vi "MAIN.vi"() -> ()   [LabVIEW 2017]
uses:
  Main Control Functions.ctl
  TableType.ctl
  <vilib>/Utility/file.llb/Write Delimited Spreadsheet (DBL).vi
  <vilib>/Utility/file.llb/Read Delimited Spreadsheet (DBL).vi
panel:
  in  "Start":bool
  in  "Listbox":i32(listbox)
  in  "Stop":bool
  out "Time":string caption="String"
  in  "String":string
  in  "Tab Control":enum32{"Page 1", "Page 2"}(tab)
  in  "Voltage":dbl caption="Numeric"
  in  "Day Code":string caption="String"
  in  "Unit ID":i32 caption="Numeric"
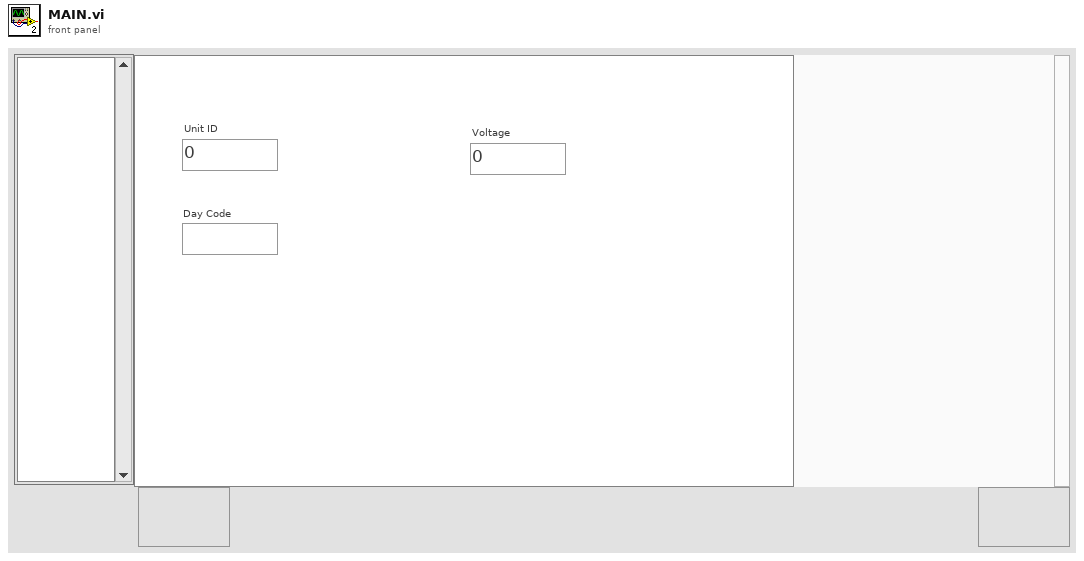
[diagram p1: front panel]
types:
  T1 = typedef "Main Control Functions.ctl" = enum16{"Initialize", "Wait", "Read PN Wfm", "Read SP Wfm", "Read FrHz Wfm", "Read FrHzV Wfm", "Read Power Wfm", "Read Curr Wfm", "Check Q", "Exit"}
  T2 = typedef "TableType.ctl" = enum16{"PhaseNoise", "Spectrum", "FreqHz", "FreqHzV", "Power", "Current"}
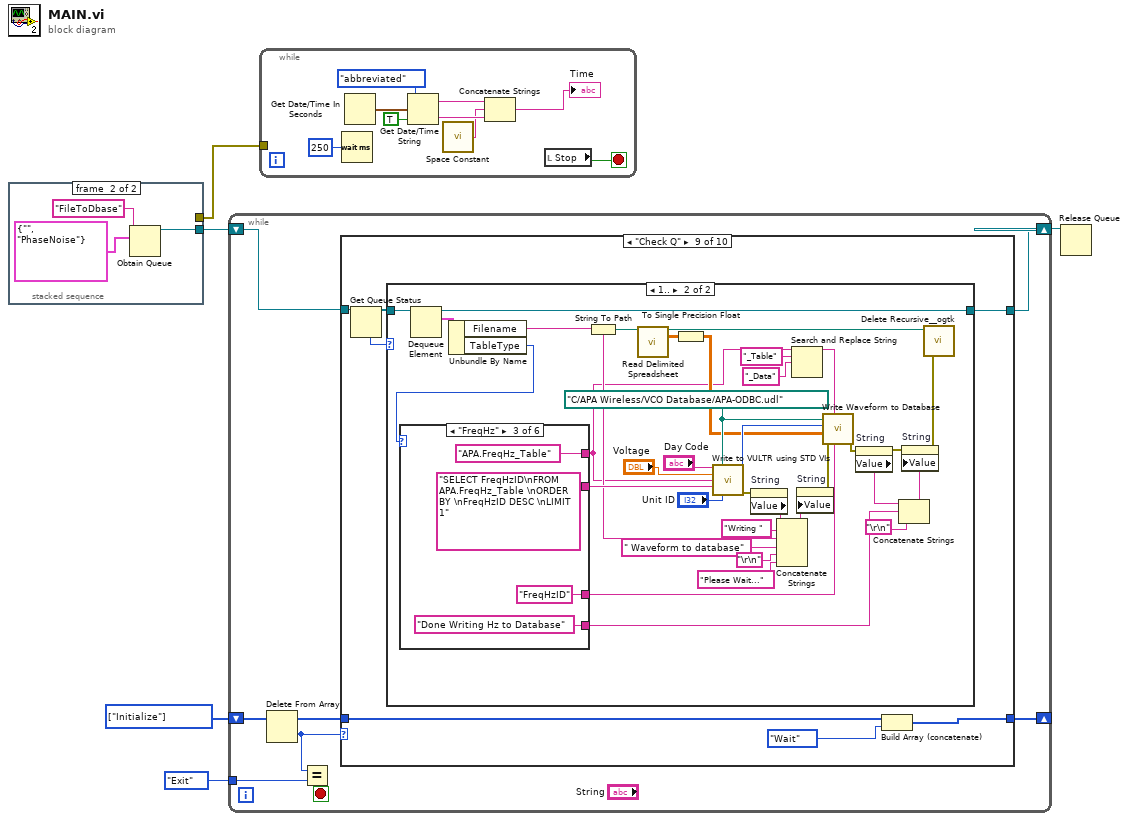
[diagram p0: block diagram]
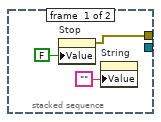
[diagram p2: hidden frame]
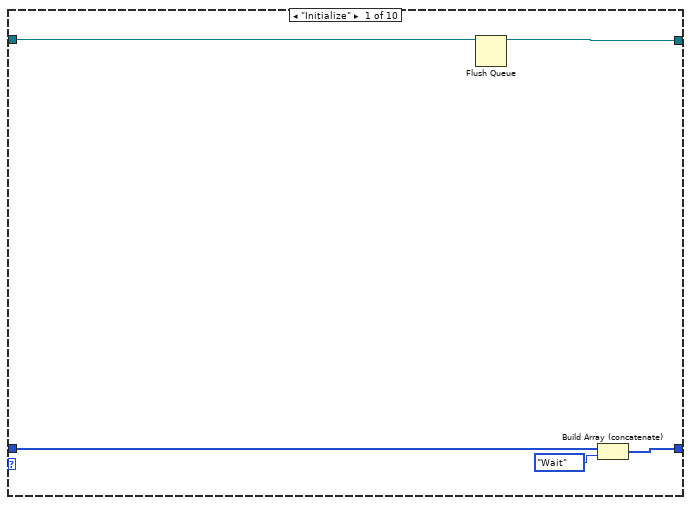
[diagram p3: hidden frame]
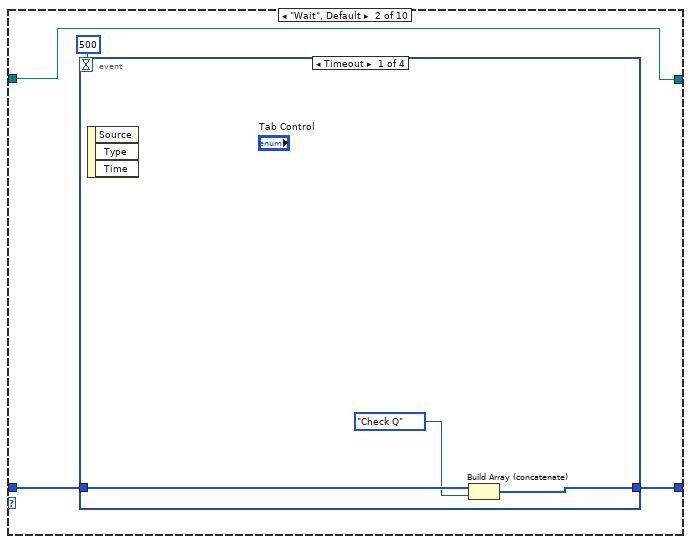
[diagram p4: hidden frame]
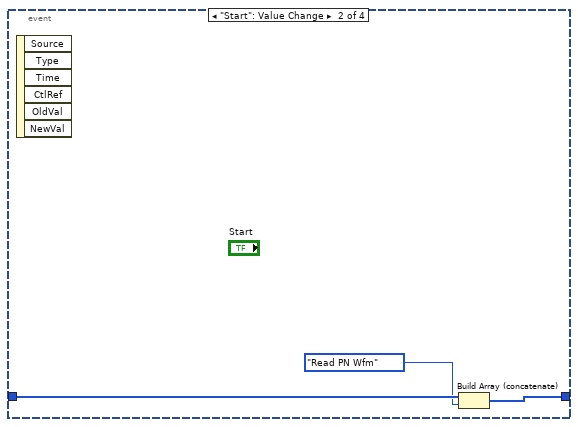
[diagram p5: hidden frame]
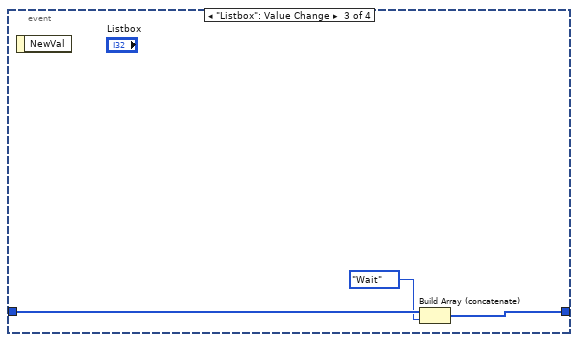
[diagram p6: hidden frame]
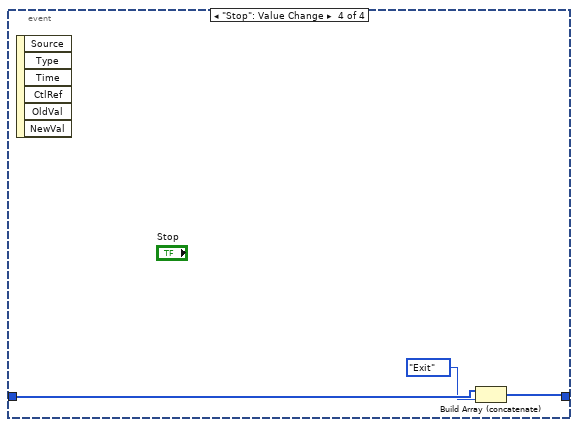
[diagram p7: hidden frame]
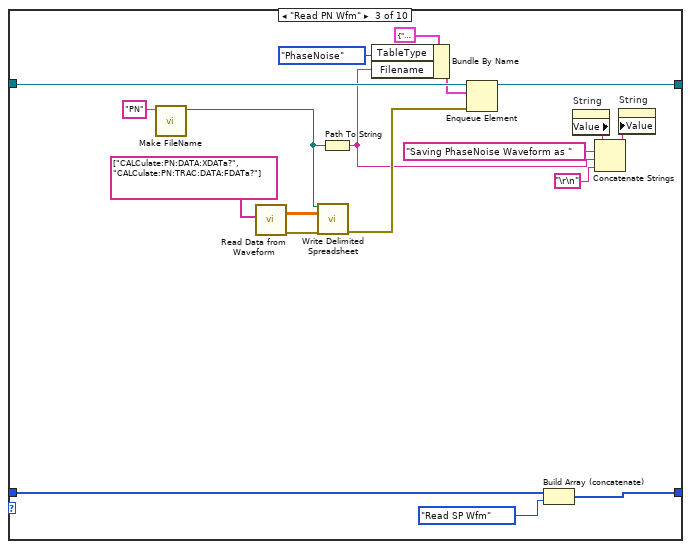
[diagram p8: hidden frame]
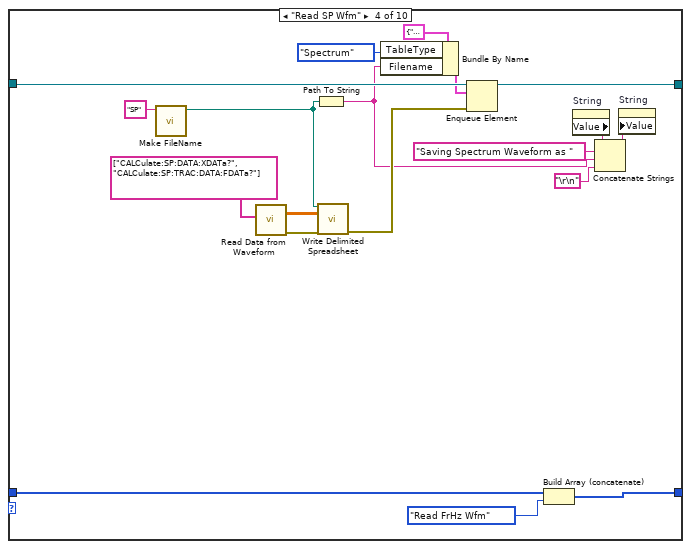
[diagram p9: hidden frame]
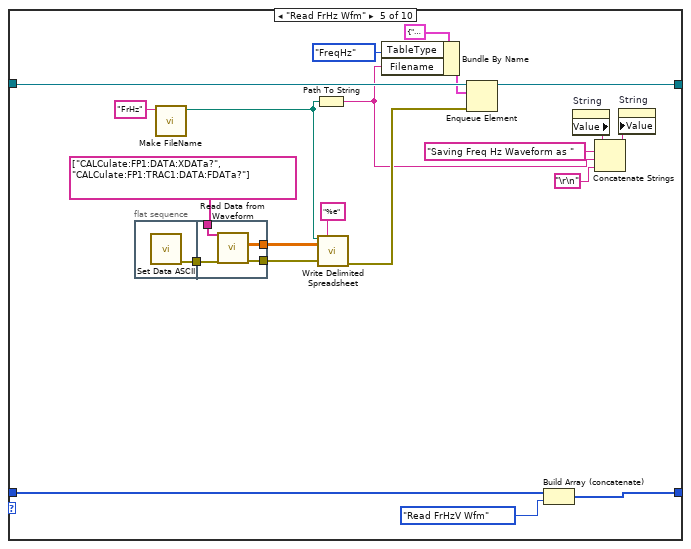
[diagram p10: hidden frame]
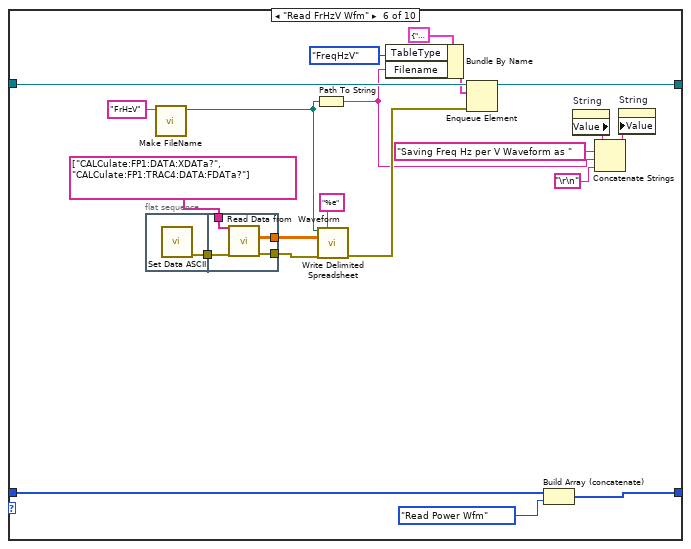
[diagram p11: hidden frame]
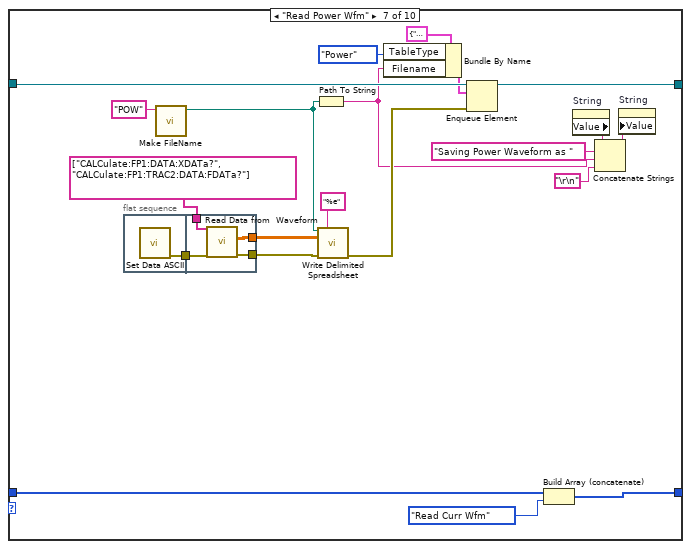
[diagram p12: hidden frame]
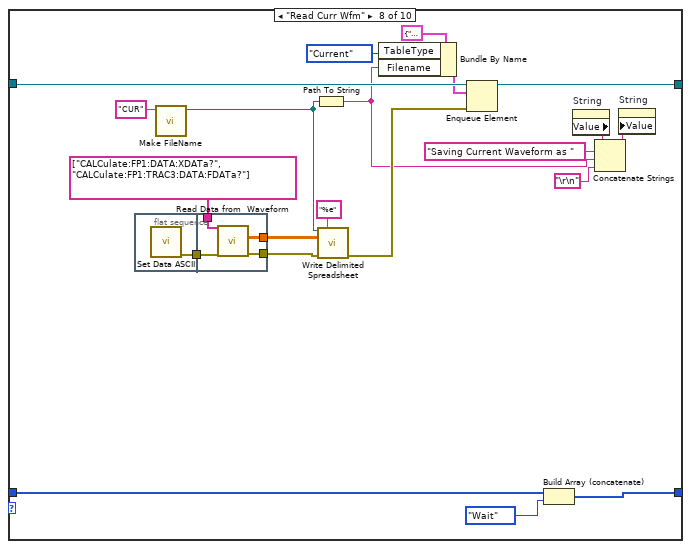
[diagram p13: hidden frame]
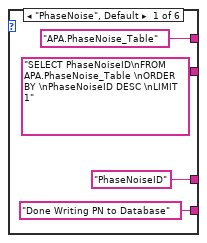
[diagram p15: hidden frame]
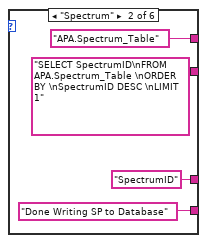
[diagram p16: hidden frame]
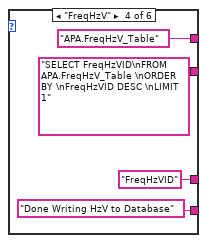
[diagram p17: hidden frame]
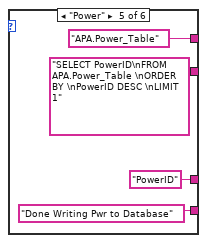
[diagram p18: hidden frame]
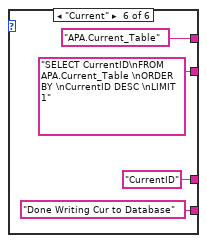
[diagram p19: hidden frame]
diagram:
  w1 = T1[] [enum."Initialize"] items=["Initialize", "Wait", "Read PN Wfm", "Read SP Wfm", "Read FrHz Wfm", "Read FrHzV Wfm", "Read Power Wfm", "Read Curr Wfm", "Check Q", "Exit"]
  n1 = stacked-sequence {
    tunnel: [_ w10] -> w3
    tunnel: [w8 _] -> w2
    frame #0 {
      n2 = property on="Stop" class="Bool (strict)"("Value"=FALSE ("Stop")) -> (error out=w8:errorcluster)  [unwired: 2 in, 1 out]
      n3 = property on="String" class="Str"("Value"="") -> ()  [unwired: 2 in, 2 out]
    }
    frame #1 {
      n4 = Obtain Queue(name (unnamed)="FileToDbase", element data type=cluster{"Filename":string, "TableType":T2} {"Filename"="", "TableType"=enum."PhaseNoise"}) -> (queue out=w10:refnum<queue>)  [unwired: 3 in, 2 out]
    }
  }
  n5 = while {
    shift-right: [w14] -> _
    shift-left: w1 -> [w17]
    tunnel: Main_Control_Functions."Exit" ("Enum") -> [w19]
    shift-right: [w12] -> w4
    shift-left: w3 -> [w13]
    stop <- w18 stop-if-true
    n6 = Delete From Array(array=w17) -> (deleted portion=w16:T1, array with subset deleted=w15:T1[])  [unwired: 2 in]
    n7 = Equal?(x=w16, y=w19) -> (x = y?=w18:bool)
    n8 = case shown="\"Check Q\"" w16 {
      tunnel: w15 -> [w24 w28 w52 w71 w95 w121 w147 w173 w189 w251]
      tunnel: [w22 w27 w47 w66 w90 w116 w142 w168 w185 w251] -> w14
      tunnel: w13 -> [w21 w26 w55 w74 w98 w124 w150 w176 w188 w250]
      tunnel: [w20 w26 w54 w73 w97 w123 w149 w175 w186 w250] -> w12
      frame "Initialize" {
        n9 = Flush Queue(queue=w21) -> (queue out=w20:refnum<queue>)  [unwired: 1 in, 2 out]
        n10 = Build Array (concatenate)(w24, Main_Control_Functions."Wait" ("Enum")) -> (w22:T1[])
      }
      frame "Wait", Default {
        n11 = event shown="[0] Timeout" {
          selector: _ -> [_ _ _ _]
          dyn-events: _ -> [_ _ _ _]
          timeout: 500 -> [_ _ _ _]
          tunnel: [w30 w33 w36 w39] -> w27
          tunnel: w28 -> [w31 w34 w37 w40]
          event Timeout {
            n12 = event-data() -> ()  [unwired: 1 in, 3 out]
            n13 = Build Array (concatenate)(w31, Main_Control_Functions."Check Q" ("Enum")) -> (w30:T1[])
          }
          event "Start": Value Change {
            n14 = event-data() -> ()  [unwired: 1 in, 6 out]
            n15 = Build Array (concatenate)(w34, Main_Control_Functions."Read PN Wfm" ("Enum")) -> (w33:T1[])
          }
          event "Listbox": Value Change {
            n16 = event-data() -> ()  [unwired: 1 in, 1 out]
            n17 = Build Array (concatenate)(w37, Main_Control_Functions."Wait" ("Enum")) -> (w36:T1[])
          }
          event "Stop": Value Change {
            n18 = event-data() -> ()  [unwired: 1 in, 6 out]
            n19 = Build Array (concatenate)(w40, Main_Control_Functions."Exit" ("Enum")) -> (w39:T1[])
          }
        }
      }
      frame "Read PN Wfm" {
        n20 = call "Make FileName.vi"("Meas Name"="PN") -> ("Path"=w56:path)  [unwired: 10 in]
        n21 = call "Read Data from  Waveform.vi"("Commands"=string[] ["CALCulate:PN:DATA:XDATa?", "CALCulate:PN:TRAC:DATA:FDATa?"]) -> ("error out"=w58:errorcluster, "Results"=w57:sgl[][])  [unwired: 9 in]
        n22 = call-poly <vilib>:"Write Delimited Spreadsheet.vi"("file path (dialog if empty)"=w56, "2D data"=w57, "error in (no error)"=w58) -> ("error out"=w53:errorcluster)  [unwired: 11 in, 1 out]
        n23 = Path To String(path=w56) -> (string=w43:string)
        n24 = Bundle By Name(cluster=cluster{"Filename":string, "TableType":T2} {"Filename"="", "TableType"=enum."PhaseNoise"} ("element"), "TableType"=TableType."PhaseNoise", "Filename"=w43) -> (w41:cluster{"Filename":string, "TableType":T2})
        n25 = Enqueue Element(queue=w55, element=w41, error in (no error)=w53) -> (queue out=w54:refnum<queue>)  [unwired: 1 in, 2 out]
        n26 = Build Array (concatenate)(w52, Main_Control_Functions."Read SP Wfm" ("Enum")) -> (w47:T1[])
        n27 = property on="String" class="Str"() -> ("Value"=w50:string)  [unwired: 2 in, 2 out]
        n28 = Concatenate Strings(w50, "Saving PhaseNoise Waveform as " ("string"), w43, "\r\n") -> (w51:string)
        n29 = property on="String" class="Str"("Value"=w51) -> ()  [unwired: 2 in, 2 out]
      }
      frame "Read SP Wfm" {
        n30 = call "Make FileName.vi"("Meas Name"="SP") -> ("Path"=w75:path)  [unwired: 10 in]
        n31 = call "Read Data from  Waveform.vi"("Commands"=string[] ["CALCulate:SP:DATA:XDATa?", "CALCulate:SP:TRAC:DATA:FDATa?"]) -> ("error out"=w77:errorcluster, "Results"=w76:sgl[][])  [unwired: 9 in]
        n32 = Path To String(path=w75) -> (string=w61:string)
        n33 = call-poly <vilib>:"Write Delimited Spreadsheet.vi"("file path (dialog if empty)"=w75, "2D data"=w76, "error in (no error)"=w77) -> ("error out"=w72:errorcluster)  [unwired: 11 in, 1 out]
        n34 = Bundle By Name(cluster=cluster{"Filename":string, "TableType":T2} {"Filename"="", "TableType"=enum."PhaseNoise"} ("element"), "TableType"=TableType."Spectrum", "Filename"=w61) -> (w60:cluster{"Filename":string, "TableType":T2})
        n35 = Enqueue Element(queue=w74, element=w60, error in (no error)=w72) -> (queue out=w73:refnum<queue>)  [unwired: 1 in, 2 out]
        n36 = Build Array (concatenate)(w71, Main_Control_Functions."Read FrHz Wfm" ("Enum")) -> (w66:T1[])
        n37 = property on="String" class="Str"() -> ("Value"=w69:string)  [unwired: 2 in, 2 out]
        n38 = Concatenate Strings(w69, "Saving Spectrum Waveform as " ("string"), w61, "\r\n") -> (w70:string)
        n39 = property on="String" class="Str"("Value"=w70) -> ()  [unwired: 2 in, 2 out]
      }
      frame "Read FrHz Wfm" {
        n40 = flat-sequence {
          tunnel: [w100] -> w87
          tunnel: w87 -> [w104]
          tunnel: string[] ["CALCulate:FP1:DATA:XDATa?", "CALCulate:FP1:TRAC1:DATA:FDATa?"] ("Commands") -> [w103]
          tunnel: [w102] -> w85
          tunnel: [w101] -> w84
          frame #0 {
            n41 = call "Set Data ASCII.vi"() -> ("error out"=w100:errorcluster)  [unwired: 11 in]
          }
          frame #1 {
            n42 = call "Read Data from  Waveform.vi"("error in (no error)"=w104, "Commands"=w103) -> ("error out"=w102:errorcluster, "Results"=w101:sgl[][])  [unwired: 8 in]
          }
        }
        n43 = call "Make FileName.vi"("Meas Name"="FrHz") -> ("Path"=w99:path)  [unwired: 10 in]
        n44 = Path To String(path=w99) -> (string=w79:string)
        n45 = call-poly <vilib>:"Write Delimited Spreadsheet.vi"("file path (dialog if empty)"=w99, "format (%.3f)"="%e", "2D data"=w84, "error in (no error)"=w85) -> ("error out"=w96:errorcluster)  [unwired: 10 in, 1 out]
        n46 = Bundle By Name(cluster=cluster{"Filename":string, "TableType":T2} {"Filename"="", "TableType"=enum."PhaseNoise"} ("element"), "TableType"=TableType."FreqHz", "Filename"=w79) -> (w80:cluster{"Filename":string, "TableType":T2})
        n47 = Enqueue Element(queue=w98, element=w80, error in (no error)=w96) -> (queue out=w97:refnum<queue>)  [unwired: 1 in, 2 out]
        n48 = Build Array (concatenate)(w95, Main_Control_Functions."Read FrHzV Wfm" ("Enum")) -> (w90:T1[])
        n49 = property on="String" class="Str"() -> ("Value"=w93:string)  [unwired: 2 in, 2 out]
        n50 = Concatenate Strings(w93, "Saving Freq Hz Waveform as " ("string"), w79, "\r\n") -> (w94:string)
        n51 = property on="String" class="Str"("Value"=w94) -> ()  [unwired: 2 in, 2 out]
      }
      frame "Read FrHzV Wfm" {
        n52 = flat-sequence {
          tunnel: [w126] -> w113
          tunnel: w113 -> [w130]
          tunnel: string[] ["CALCulate:FP1:DATA:XDATa?", "CALCulate:FP1:TRAC4:DATA:FDATa?"] ("Commands") -> [w129]
          tunnel: [w128] -> w110
          tunnel: [w127] -> w111
          frame #0 {
            n53 = call "Set Data ASCII.vi"() -> ("error out"=w126:errorcluster)  [unwired: 11 in]
          }
          frame #1 {
            n54 = call "Read Data from  Waveform.vi"("error in (no error)"=w130, "Commands"=w129) -> ("error out"=w128:errorcluster, "Results"=w127:sgl[][])  [unwired: 8 in]
          }
        }
        n55 = call "Make FileName.vi"("Meas Name"="FrHzV") -> ("Path"=w125:path)  [unwired: 10 in]
        n56 = Path To String(path=w125) -> (string=w105:string)
        n57 = call-poly <vilib>:"Write Delimited Spreadsheet.vi"("file path (dialog if empty)"=w125, "format (%.3f)"="%e", "2D data"=w111, "error in (no error)"=w110) -> ("error out"=w122:errorcluster)  [unwired: 10 in, 1 out]
        n58 = Bundle By Name(cluster=cluster{"Filename":string, "TableType":T2} {"Filename"="", "TableType"=enum."PhaseNoise"} ("element"), "TableType"=TableType."FreqHzV", "Filename"=w105) -> (w106:cluster{"Filename":string, "TableType":T2})
        n59 = Enqueue Element(queue=w124, element=w106, error in (no error)=w122) -> (queue out=w123:refnum<queue>)  [unwired: 1 in, 2 out]
        n60 = Build Array (concatenate)(w121, Main_Control_Functions."Read Power Wfm" ("Enum")) -> (w116:T1[])
        n61 = property on="String" class="Str"() -> ("Value"=w119:string)  [unwired: 2 in, 2 out]
        n62 = Concatenate Strings(w119, "Saving Freq Hz per V Waveform as " ("string"), w105, "\r\n") -> (w120:string)
        n63 = property on="String" class="Str"("Value"=w120) -> ()  [unwired: 2 in, 2 out]
      }
      frame "Read Power Wfm" {
        n64 = flat-sequence {
          tunnel: [w152] -> w139
          tunnel: w139 -> [w156]
          tunnel: string[] ["CALCulate:FP1:DATA:XDATa?", "CALCulate:FP1:TRAC2:DATA:FDATa?"] ("Commands") -> [w155]
          tunnel: [w154] -> w137
          tunnel: [w153] -> w138
          frame #0 {
            n65 = call "Set Data ASCII.vi"() -> ("error out"=w152:errorcluster)  [unwired: 11 in]
          }
          frame #1 {
            n66 = call "Read Data from  Waveform.vi"("error in (no error)"=w156, "Commands"=w155) -> ("error out"=w154:errorcluster, "Results"=w153:sgl[][])  [unwired: 8 in]
          }
        }
        n67 = call "Make FileName.vi"("Meas Name"="POW") -> ("Path"=w151:path)  [unwired: 10 in]
        n68 = Path To String(path=w151) -> (string=w131:string)
        n69 = call-poly <vilib>:"Write Delimited Spreadsheet.vi"("file path (dialog if empty)"=w151, "format (%.3f)"="%e", "2D data"=w138, "error in (no error)"=w137) -> ("error out"=w148:errorcluster)  [unwired: 10 in, 1 out]
        n70 = Bundle By Name(cluster=cluster{"Filename":string, "TableType":T2} {"Filename"="", "TableType"=enum."PhaseNoise"} ("element"), "TableType"=TableType."Power", "Filename"=w131) -> (w132:cluster{"Filename":string, "TableType":T2})
        n71 = Enqueue Element(queue=w150, element=w132, error in (no error)=w148) -> (queue out=w149:refnum<queue>)  [unwired: 1 in, 2 out]
        n72 = Build Array (concatenate)(w147, Main_Control_Functions."Read Curr Wfm" ("Enum")) -> (w142:T1[])
        n73 = property on="String" class="Str"() -> ("Value"=w145:string)  [unwired: 2 in, 2 out]
        n74 = Concatenate Strings(w145, "Saving Power Waveform as " ("string"), w131, "\r\n") -> (w146:string)
        n75 = property on="String" class="Str"("Value"=w146) -> ()  [unwired: 2 in, 2 out]
      }
      frame "Read Curr Wfm" {
        n76 = flat-sequence {
          tunnel: [w178] -> w165
          tunnel: w165 -> [w182]
          tunnel: string[] ["CALCulate:FP1:DATA:XDATa?", "CALCulate:FP1:TRAC3:DATA:FDATa?"] ("Commands") -> [w181]
          tunnel: [w180] -> w163
          tunnel: [w179] -> w164
          frame #0 {
            n77 = call "Set Data ASCII.vi"() -> ("error out"=w178:errorcluster)  [unwired: 11 in]
          }
          frame #1 {
            n78 = call "Read Data from  Waveform.vi"("error in (no error)"=w182, "Commands"=w181) -> ("error out"=w180:errorcluster, "Results"=w179:sgl[][])  [unwired: 8 in]
          }
        }
        n79 = call "Make FileName.vi"("Meas Name"="CUR") -> ("Path"=w177:path)  [unwired: 10 in]
        n80 = Path To String(path=w177) -> (string=w157:string)
        n81 = call-poly <vilib>:"Write Delimited Spreadsheet.vi"("file path (dialog if empty)"=w177, "format (%.3f)"="%e", "2D data"=w164, "error in (no error)"=w163) -> ("error out"=w174:errorcluster)  [unwired: 10 in, 1 out]
        n82 = Bundle By Name(cluster=cluster{"Filename":string, "TableType":T2} {"Filename"="", "TableType"=enum."PhaseNoise"} ("element"), "TableType"=TableType."Current", "Filename"=w157) -> (w158:cluster{"Filename":string, "TableType":T2})
        n83 = Enqueue Element(queue=w176, element=w158, error in (no error)=w174) -> (queue out=w175:refnum<queue>)  [unwired: 1 in, 2 out]
        n84 = Build Array (concatenate)(w173, Main_Control_Functions."Wait" ("Enum")) -> (w168:T1[])
        n85 = property on="String" class="Str"() -> ("Value"=w171:string)  [unwired: 2 in, 2 out]
        n86 = Concatenate Strings(w171, "Saving Current Waveform as " ("string"), w157, "\r\n") -> (w172:string)
        n87 = property on="String" class="Str"("Value"=w172) -> ()  [unwired: 2 in, 2 out]
      }
      frame "Check Q" {
        n88 = Get Queue Status(queue=w188) -> (queue out=w187:refnum<queue>, # elements in queue=w183:i32)  [unwired: 2 in, 6 out]
        n89 = case shown="1.." w183 {
          tunnel: w187 -> [w190 w225]
          tunnel: [w190 w220] -> w186
          frame ..0 {
          }
          frame 1.. {
            w204 = path "C:/APA Wireless/VCO Database/APA-ODBC.udl" ("conninfo")
            n90 = Dequeue Element(queue=w225) -> (queue out=w220:refnum<queue>, element=w198:cluster{"Filename":string, "TableType":T2})  [unwired: 2 in, 2 out]
            n91 = Unbundle By Name(w198) -> ("Filename"=w197:string, "TableType"=w196:T2)
            n92 = case shown="\"FreqHz\"" w196 {
              tunnel: ["Done Writing PN to Database" ("string") "Done Writing SP to Database" ("string") "Done Writing Hz to Database" ("string") "Done Writing HzV to Database" ("string") "Done Writing Pwr to Database" ("string") "Done Writing Cur to Database" ("string")] -> w207
              tunnel: ["SELECT PhaseNoiseID\nFROM APA.PhaseNoise_Table \nORDER BY \nPhaseNoiseID DESC \nLIMIT 1" ("SQL query") "SELECT SpectrumID\nFROM APA.Spectrum_Table \nORDER BY \nSpectrumID DESC \nLIMIT 1" ("SQL query") "SELECT FreqHzID\nFROM APA.FreqHz_Table \nORDER BY \nFreqHzID DESC \nLIMIT 1" ("SQL query") "SELECT FreqHzVID\nFROM APA.FreqHzV_Table \nORDER BY \nFreqHzVID DESC \nLIMIT 1" ("SQL query") "SELECT PowerID\nFROM APA.Power_Table \nORDER BY \nPowerID DESC \nLIMIT 1" ("SQL query") "SELECT CurrentID\nFROM APA.Current_Table \nORDER BY \nCurrentID DESC \nLIMIT 1" ("SQL query")] -> w200
              tunnel: ["APA.PhaseNoise_Table" ("Table") "APA.Spectrum_Table" ("Table") "APA.FreqHz_Table" ("Table") "APA.FreqHzV_Table" ("Table") "APA.Power_Table" ("Table") "APA.Current_Table" ("Table")] -> w194
              tunnel: ["PhaseNoiseID" ("Field") "SpectrumID" ("Field") "FreqHzID" ("Field") "FreqHzVID" ("Field") "PowerID" ("Field") "CurrentID" ("Field")] -> w195
              frame "PhaseNoise", Default {
              }
              frame "Spectrum" {
              }
              frame "FreqHz" {
              }
              frame "FreqHzV" {
              }
              frame "Power" {
              }
              frame "Current" {
              }
            }
            n93 = String To Path(string=w197) -> (path=w202:path)
            n94 = call-poly <vilib>:"Read Delimited Spreadsheet.vi"("file path (dialog if empty)"=w202) -> ("new file path (Not A Path if cancelled)"=w201:path, "all rows"=w219:dbl[][])  [unwired: 9 in, 4 out]
            n95 = To Single Precision Float(number=w219) -> (single precision float=w199:sgl[][])
            n96 = call "Write to VULTR using STD VIs.vi"("DayCode"="Day Code", "conninfo"=w204, "Voltage"="Voltage", "Table"=w194, "SQL query"=w200, "UnitID"="Unit ID") -> ("Get ID"=w221:i32, "error out"=w215:errorcluster)  [unwired: 8 in]
            n97 = property on="String" class="Str"(error in=w215) -> ("Value"=w217:string)  [unwired: 1 in, 2 out]
            n98 = Concatenate Strings(w217, "Writing " ("string"), w197, " Waveform to database" ("string"), "\r\n", "Please Wait...") -> (w218:string)
            n99 = Search and Replace String(input string=w194, search string="_Table", replace string="_Data" ("search string")) -> (result string=w193:string)  [unwired: 5 in, 3 out]
            n100 = property on="String" class="Str"("Value"=w218) -> (error out=w212:errorcluster)  [unwired: 2 in, 1 out]
            n101 = call "Write Waveform to Database.vi"("Field"=w195, "Table"=w193, "error in (no error)"=w212, "Array"=w199, "FreqID"=w221, "conninfo"=w204) -> ("error out"=w210:errorcluster)  [unwired: 5 in]
            n102 = property on="String" class="Str"(error in=w210) -> (error out=w203:errorcluster, "Value"=w208:string)  [unwired: 1 in, 1 out]
            n103 = Concatenate Strings(w208, w207, "\r\n") -> (w209:string)
            n104 = property on="String" class="Str"(error in=w203, "Value"=w209) -> (error out=w205:errorcluster)  [unwired: 1 in, 1 out]
            n105 = call <userlib>:"Delete Recursive__ogtk.vi"("error in (no error)"=w205, "Path"=w201) -> ()  [unwired: 8 in, 2 out]
          }
        }
        n106 = Build Array (concatenate)(w189, Main_Control_Functions."Wait" ("Enum")) -> (w185:T1[])
      }
      frame "Exit" {
      }
    }
  }
  n107 = while {
    tunnel: w2 -> [_]
    stop <- w254 stop-if-true
    n108 = Wait (ms)(milliseconds to wait=u32 250) -> ()  [unwired: 1 out]
    n109 = Get Date/Time In Seconds() -> (seconds since 1Jan1904=w252:timestamp)
    n110 = Get Date/Time String(date format (0)=enum16{"short", "long", "abbreviated"}."abbreviated", seconds (now)=w252, want seconds? (F)=TRUE) -> (date string=w258:string, time string=w257:string)
    n111 = call <vilib>:"Space Constant.vi"() -> ("String"=w256:string)
    n112 = Concatenate Strings(w258, w256, w257) -> (→"Time":string)
    n113 = local read "Stop"() -> (w254:bool)
  }
  n114 = Release Queue(queue=w4) -> ()  [unwired: 2 in, 3 out]
